vi "DCmotorHbridge.vi"() -> ()   [LabVIEW 2020]
uses:
  Control 1.ctl
  <vilib>/DAQmx/create/channels.llb/DAQmx Create Channel (CO-Pulse Generation-Frequency).vi
  <vilib>/DAQmx/configure/timing.llb/DAQmx Timing (Implicit).vi
  <resource>/objmgr/daqmx.rc
panel:
  in  "Motor Stop":bool
  in  "Direction":bool
  in  "Motor Start":bool
  in  "Speed":dbl(knob) scale=0.01..0.99
  in  "Output B":tag
  in  "Output A":tag
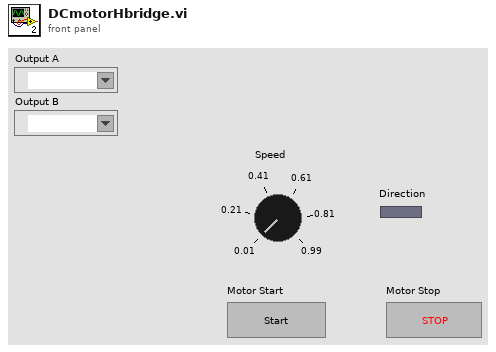
[diagram p1: front panel]
types:
  T1 = typedef "Control 1.ctl" = enum16{"Idle", "Change Direction", "Change Speed", "Start", "Stop"}
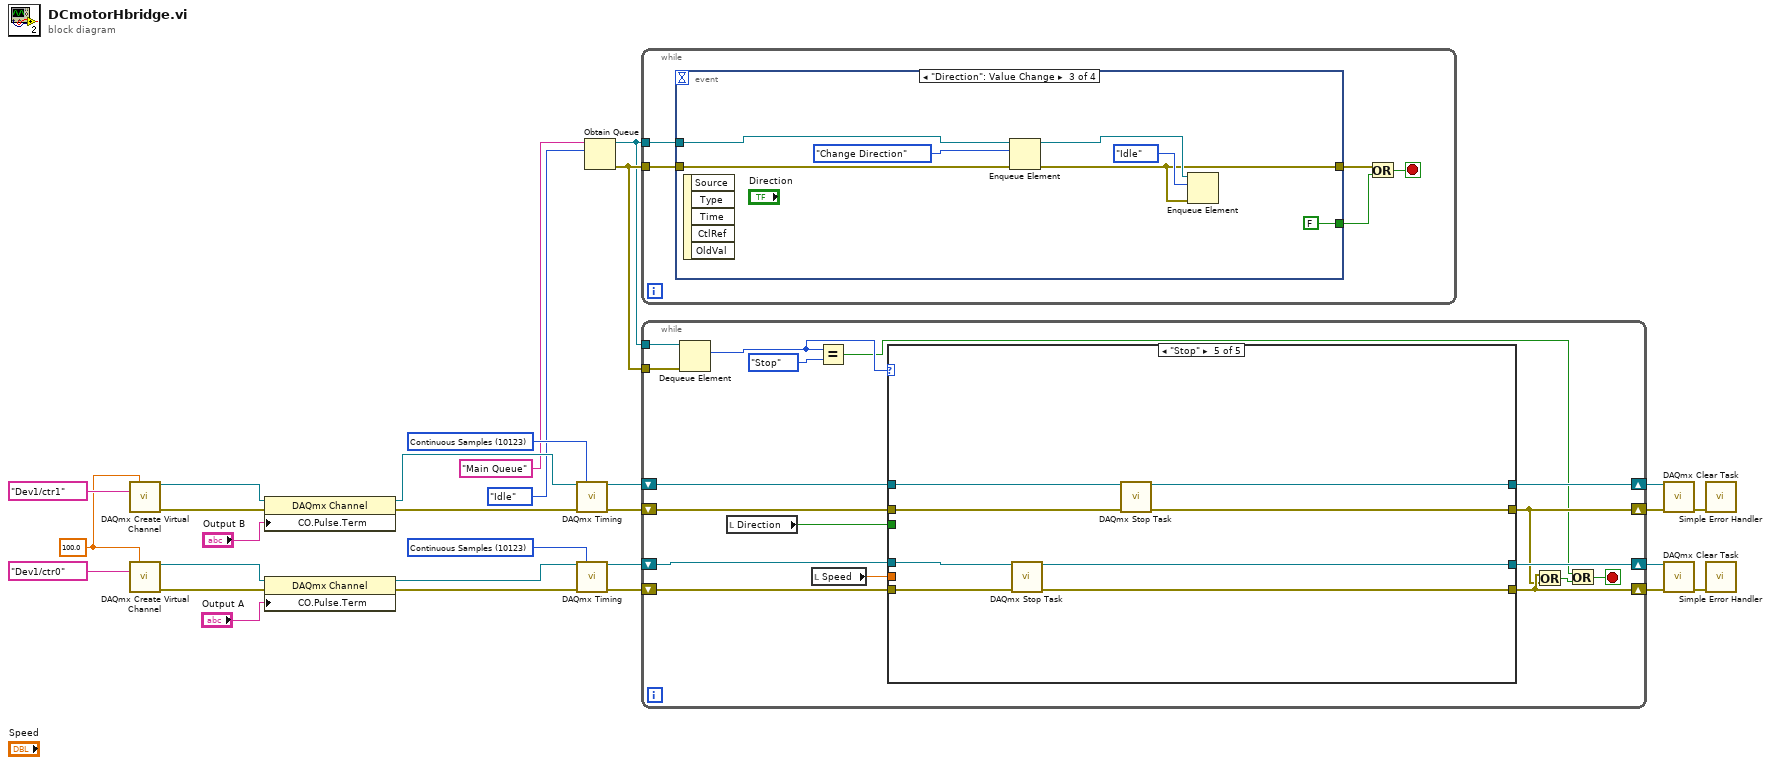
[diagram p0: block diagram]
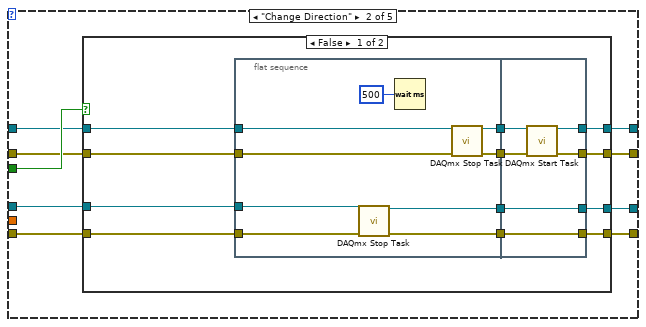
[diagram p3: hidden frame]
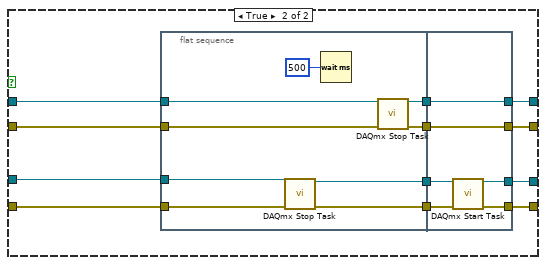
[diagram p4: hidden frame]
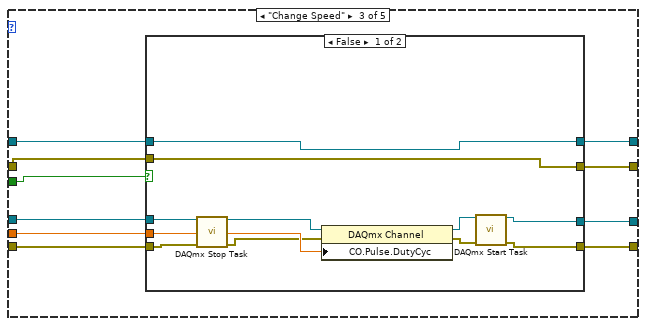
[diagram p5: hidden frame]
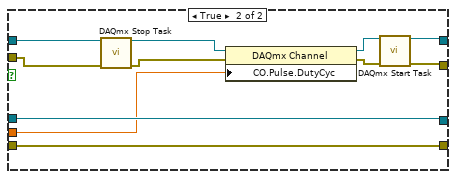
[diagram p6: hidden frame]
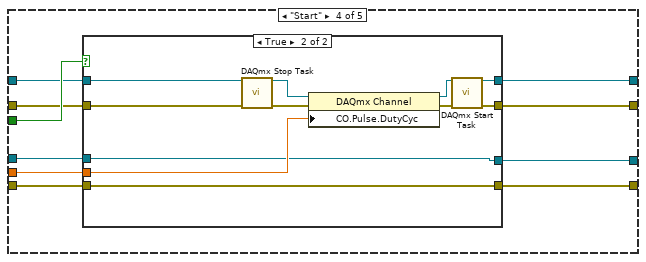
[diagram p7: hidden frame]
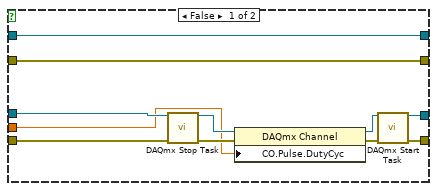
[diagram p8: hidden frame]
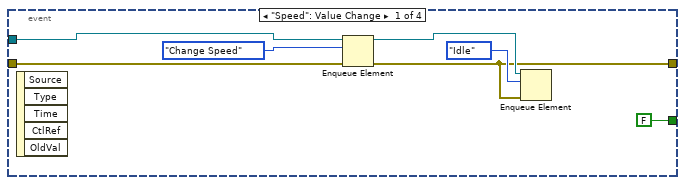
[diagram p9: hidden frame]
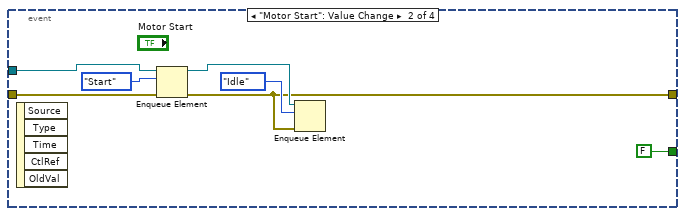
[diagram p10: hidden frame]
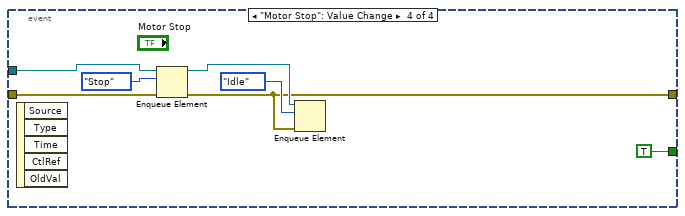
[diagram p11: hidden frame]
diagram:
  w1 = 100.0 ("frequency")
  w16 = 10123 items=["Finite Samples"=10178, "Continuous Samples"=10123, "Hardware Timed Single Point"=12522] ("sample mode")
  w17 = 10123 items=["Finite Samples"=10178, "Continuous Samples"=10123, "Hardware Timed Single Point"=12522] ("sample mode")
  n1 = call-poly <vilib>:"DAQmx Create Virtual Channel.vi"("frequency"=w1, "counter"=tag "Dev1/ctr1") -> ("task out"=w29:refnum<k21>, "error out"=w28:errorcluster)  [unwired: 12 in]
  n2 = call-poly <vilib>:"DAQmx Create Virtual Channel.vi"("frequency"=w1, "counter"=tag "Dev1/ctr0") -> ("task out"=w26:refnum<k21>, "error out"=w27:errorcluster)  [unwired: 12 in]
  n3 = property class="DAQmx Channel"(reference=w29, error in=w28, "CO.Pulse.Term"="Output B") -> (reference out=w19:refnum<k21>, error out=w18:errorcluster)
  n4 = property class="DAQmx Channel"(reference=w26, error in=w27, "CO.Pulse.Term"="Output A") -> (reference out=w21:refnum<k21>, error out=w20:errorcluster)
  n5 = call-poly <vilib>:"DAQmx Timing.vi"("task/channels in"=w19, "sample mode"=w16, "error in"=w18) -> ("task out"=w13:refnum<k21>, "error out"=w12:errorcluster)  [unwired: 11 in]
  n6 = call-poly <vilib>:"DAQmx Timing.vi"("task/channels in"=w21, "sample mode"=w17, "error in"=w20) -> ("task out"=w11:refnum<k21>, "error out"=w10:errorcluster)  [unwired: 11 in]
  n7 = Obtain Queue(name (unnamed)="Main Queue", element data type=Control_1."Idle") -> (queue out=w6:refnum<queue>, error out=w7:errorcluster)  [unwired: 3 in, 1 out]
  n8 = while {
    tunnel: w7 -> [w33]
    tunnel: w6 -> [w34]
    stop <- w31 stop-if-true
    n9 = event shown="[2] \"Direction\": Value Change" {
      selector: _ -> [_ _ _ _]
      dyn-events: _ -> [_ _ _ _]
      timeout: _ -> [_ _ _ _]
      tunnel: w34 -> [w41 w45 w52 w59]
      tunnel: w33 -> [w40 w44 w51 w58]
      tunnel: [w36 w43 w50 w57] -> w30
      tunnel: [FALSE FALSE FALSE TRUE] -> w32
      event "Speed": Value Change {
        n10 = event-data() -> ()  [unwired: 1 in, 5 out]
        n11 = Enqueue Element(queue=w41, element=Control_1."Change Speed", error in (no error)=w40) -> (queue out=w38:refnum<queue>, error out=w36:errorcluster)  [unwired: 1 in, 1 out]
        n12 = Enqueue Element(queue=w38, element=Control_1."Idle", error in (no error)=w36) -> ()  [unwired: 1 in, 3 out]
      }
      event "Motor Start": Value Change {
        n13 = event-data() -> ()  [unwired: 1 in, 5 out]
        n14 = Enqueue Element(queue=w45, element=Control_1."Start", error in (no error)=w44) -> (queue out=w47:refnum<queue>, error out=w43:errorcluster)  [unwired: 1 in, 1 out]
        n15 = Enqueue Element(queue=w47, element=Control_1."Idle", error in (no error)=w43) -> ()  [unwired: 1 in, 3 out]
      }
      event "Direction": Value Change {
        n16 = event-data() -> ()  [unwired: 1 in, 5 out]
        n17 = Enqueue Element(queue=w52, element=Control_1."Change Direction", error in (no error)=w51) -> (queue out=w55:refnum<queue>, error out=w50:errorcluster)  [unwired: 1 in, 1 out]
        n18 = Enqueue Element(queue=w55, element=Control_1."Idle", error in (no error)=w50) -> ()  [unwired: 1 in, 3 out]
      }
      event "Motor Stop": Value Change {
        n19 = event-data() -> ()  [unwired: 1 in, 5 out]
        n20 = Enqueue Element(queue=w59, element=Control_1."Stop", error in (no error)=w58) -> (queue out=w61:refnum<queue>, error out=w57:errorcluster)  [unwired: 1 in, 1 out]
        n21 = Enqueue Element(queue=w61, element=Control_1."Idle", error in (no error)=w57) -> ()  [unwired: 1 in, 3 out]
      }
    }
    n22 = Or(x=w30, y=w32) -> (x .or. y?=w31:bool)
  }
  n23 = while {
    tunnel: w6 -> [w71]
    shift-right: [w68] -> w4
    shift-left: w12 -> [w78]
    shift-right: [w75] -> w5
    shift-left: w13 -> [w79]
    shift-right: [w74] -> w3
    shift-left: w11 -> [w77]
    shift-right: [w69] -> w2
    shift-left: w10 -> [w76]
    tunnel: w7 -> [w67]
    stop <- w70 stop-if-true
    n24 = Dequeue Element(queue=w71, error in (no error)=w67) -> (element=w66:T1)  [unwired: 1 in, 3 out]
    n25 = local read "Direction"() -> (w73:bool)
    n26 = local read "Speed"() -> (w72:dbl)
    n27 = Equal?(x=w66, y=Control_1."Stop") -> (x = y?=w64:bool)
    n28 = case shown="\"Stop\"" w66 {
      tunnel: w79 -> [w83 w91 w151 w182 w218]
      tunnel: w78 -> [w82 w90 w150 w181 w217]
      tunnel: w77 -> [w81 w89 w156 w188 w216]
      tunnel: w76 -> [w80 w88 w155 w187 w215]
      tunnel: [w83 w87 w149 w180 w212] -> w75
      tunnel: [w82 w86 w148 w179 w211] -> w68
      tunnel: [w81 w85 w154 w186 w214] -> w74
      tunnel: [w80 w84 w153 w185 w213] -> w69
      tunnel: w73 -> [_ w92 w147 w183 _]
      tunnel: w72 -> [_ _ w152 w184 _]
      frame "Idle" {
      }
      frame "Change Direction" {
        n29 = case shown="False" w92 {
          tunnel: w91 -> [w100 w127]
          tunnel: w90 -> [w99 w126]
          tunnel: w89 -> [w98 w125]
          tunnel: w88 -> [w97 w124]
          tunnel: [w93 w120] -> w87
          tunnel: [w94 w123] -> w86
          tunnel: [w95 w122] -> w85
          tunnel: [w96 w121] -> w84
          frame False {
            n30 = flat-sequence {
              tunnel: w99 -> [w113]
              tunnel: w100 -> [w112]
              tunnel: [w111] -> w104
              tunnel: [w110] -> w103
              tunnel: [w109] -> w102
              tunnel: [w108] -> w101
              tunnel: w97 -> [w107]
              tunnel: w98 -> [w106]
              tunnel: w104 -> [w117]
              tunnel: w103 -> [w116]
              tunnel: w102 -> [w119]
              tunnel: w101 -> [w118]
              tunnel: [w115] -> w93
              tunnel: [w114] -> w94
              tunnel: [w119] -> w95
              tunnel: [w118] -> w96
              frame #0 {
                n31 = call <vilib>:"DAQmx Stop Task.vi"("task/channels in"=w106, "error in"=w107) -> ("task out"=w109:refnum<k21>, "error out"=w108:errorcluster)  [unwired: 12 in]
                n32 = Wait (ms)(milliseconds to wait=u32 500) -> ()  [unwired: 1 out]
                n33 = call <vilib>:"DAQmx Stop Task.vi"("task/channels in"=w112, "error in"=w113) -> ("task out"=w111:refnum<k21>, "error out"=w110:errorcluster)  [unwired: 12 in]
              }
              frame #1 {
                n34 = call <vilib>:"DAQmx Start Task.vi"("task/channels in"=w117, "error in"=w116) -> ("task out"=w115:refnum<k21>, "error out"=w114:errorcluster)  [unwired: 12 in]
              }
            }
          }
          frame True {
            n35 = flat-sequence {
              tunnel: w126 -> [w140]
              tunnel: w127 -> [w139]
              tunnel: [w138] -> w131
              tunnel: [w137] -> w130
              tunnel: [w136] -> w129
              tunnel: [w135] -> w128
              tunnel: w124 -> [w134]
              tunnel: w125 -> [w133]
              tunnel: w131 -> [w141]
              tunnel: w130 -> [w142]
              tunnel: w129 -> [w146]
              tunnel: w128 -> [w145]
              tunnel: [w141] -> w120
              tunnel: [w142] -> w123
              tunnel: [w144] -> w122
              tunnel: [w143] -> w121
              frame #0 {
                n36 = call <vilib>:"DAQmx Stop Task.vi"("task/channels in"=w133, "error in"=w134) -> ("task out"=w136:refnum<k21>, "error out"=w135:errorcluster)  [unwired: 12 in]
                n37 = Wait (ms)(milliseconds to wait=u32 500) -> ()  [unwired: 1 out]
                n38 = call <vilib>:"DAQmx Stop Task.vi"("task/channels in"=w139, "error in"=w140) -> ("task out"=w138:refnum<k21>, "error out"=w137:errorcluster)  [unwired: 12 in]
              }
              frame #1 {
                n39 = call <vilib>:"DAQmx Start Task.vi"("task/channels in"=w146, "error in"=w145) -> ("task out"=w144:refnum<k21>, "error out"=w143:errorcluster)  [unwired: 12 in]
              }
            }
          }
        }
      }
      frame "Change Speed" {
        n40 = case shown="False" w147 {
          tunnel: w156 -> [w164 w170]
          tunnel: w155 -> [w163 w169]
          tunnel: [w158 w170] -> w154
          tunnel: [w157 w169] -> w153
          tunnel: w152 -> [w167 w168]
          tunnel: w151 -> [w165 w174]
          tunnel: w150 -> [w166 w173]
          tunnel: [w165 w172] -> w149
          tunnel: [w166 w171] -> w148
          frame False {
            n41 = call <vilib>:"DAQmx Stop Task.vi"("task/channels in"=w164, "error in"=w163) -> ("task out"=w162:refnum<k21>, "error out"=w161:errorcluster)  [unwired: 12 in]
            n42 = property class="DAQmx Channel"(reference=w162, error in=w161, "CO.Pulse.DutyCyc"=w167) -> (reference out=w160:refnum<k21>, error out=w159:errorcluster)
            n43 = call <vilib>:"DAQmx Start Task.vi"("task/channels in"=w160, "error in"=w159) -> ("task out"=w158:refnum<k21>, "error out"=w157:errorcluster)  [unwired: 12 in]
          }
          frame True {
            n44 = call <vilib>:"DAQmx Stop Task.vi"("task/channels in"=w174, "error in"=w173) -> ("task out"=w175:refnum<k21>, "error out"=w176:errorcluster)  [unwired: 12 in]
            n45 = property class="DAQmx Channel"(reference=w175, error in=w176, "CO.Pulse.DutyCyc"=w168) -> (reference out=w177:refnum<k21>, error out=w178:errorcluster)
            n46 = call <vilib>:"DAQmx Start Task.vi"("task/channels in"=w177, "error in"=w178) -> ("task out"=w172:refnum<k21>, "error out"=w171:errorcluster)  [unwired: 12 in]
          }
        }
      }
      frame "Start" {
        n47 = case shown="True" w183 {
          tunnel: w188 -> [w199 w201]
          tunnel: w187 -> [w198 w200]
          tunnel: [w193 w201] -> w186
          tunnel: [w192 w200] -> w185
          tunnel: w184 -> [w191 w202]
          tunnel: w182 -> [w190 w206]
          tunnel: w181 -> [w189 w205]
          tunnel: [w190 w204] -> w180
          tunnel: [w189 w203] -> w179
          frame False {
            n48 = call <vilib>:"DAQmx Stop Task.vi"("task/channels in"=w199, "error in"=w198) -> ("task out"=w197:refnum<k21>, "error out"=w196:errorcluster)  [unwired: 12 in]
            n49 = property class="DAQmx Channel"(reference=w197, error in=w196, "CO.Pulse.DutyCyc"=w191) -> (reference out=w195:refnum<k21>, error out=w194:errorcluster)
            n50 = call <vilib>:"DAQmx Start Task.vi"("task/channels in"=w195, "error in"=w194) -> ("task out"=w193:refnum<k21>, "error out"=w192:errorcluster)  [unwired: 12 in]
          }
          frame True {
            n51 = call <vilib>:"DAQmx Stop Task.vi"("task/channels in"=w206, "error in"=w205) -> ("task out"=w207:refnum<k21>, "error out"=w208:errorcluster)  [unwired: 12 in]
            n52 = property class="DAQmx Channel"(reference=w207, error in=w208, "CO.Pulse.DutyCyc"=w202) -> (reference out=w209:refnum<k21>, error out=w210:errorcluster)
            n53 = call <vilib>:"DAQmx Start Task.vi"("task/channels in"=w209, "error in"=w210) -> ("task out"=w204:refnum<k21>, "error out"=w203:errorcluster)  [unwired: 12 in]
          }
        }
      }
      frame "Stop" {
        n54 = call <vilib>:"DAQmx Stop Task.vi"("task/channels in"=w216, "error in"=w215) -> ("task out"=w214:refnum<k21>, "error out"=w213:errorcluster)  [unwired: 12 in]
        n55 = call <vilib>:"DAQmx Stop Task.vi"("task/channels in"=w218, "error in"=w217) -> ("task out"=w212:refnum<k21>, "error out"=w211:errorcluster)  [unwired: 12 in]
      }
    }
    n56 = Or(x=w69, y=w68) -> (x .or. y?=w63:bool)
    n57 = Or(x=w64, y=w63) -> (x .or. y?=w70:bool)
  }
  n58 = call <vilib>:"DAQmx Clear Task.vi"("task in"=w5, "error in"=w4) -> ("error out"=w15:errorcluster)  [unwired: 13 in]
  n59 = call <vilib>:"DAQmx Clear Task.vi"("task in"=w3, "error in"=w2) -> ("error out"=w14:errorcluster)  [unwired: 13 in]
  n60 = call <vilib>:"Simple Error Handler.vi"("error in (no error)"=w15) -> ()  [unwired: 4 in, 5 out]
  n61 = call <vilib>:"Simple Error Handler.vi"("error in (no error)"=w14) -> ()  [unwired: 4 in, 5 out]
